vi "Main_v2.vi"() -> ()   [LabVIEW 2018, in "Application.lvlib"]
doc: "This VI is the main application VI in the Delacor QMH project template. This application VI is implemented as a simple state machine, which communicates with two different Delacor QMH modules.\n_____\nBased on DQMH Project Template 6.0.0.91."
uses:
  Application.lvlib
  type defs/HW config.ctl
  eMIC response.ctl
  Application Data--cluster.ctl
  DRV cluster.ctl
  App States.ctl
  eMICs Cluster.ctl
  Switches Module/MB switches Module.lvlib
  CE14 eMIC module/CE14 eMIC module.lvlib
  MB 01 switches Module/MB 01 switches Module.lvlib
  DMM Module/DMM Module.lvlib
  CE14  Module/CE14  Module.lvlib
panel:
  out "eMIC response":T1
  out "HV60D button":refnum<vi>[](array[refnum])
  out "HW config":T2={"DMM"="COM15", "mux"="COM11", "demux"="COM16", "eMIC1"="COM13", "eMIC2"="COM6", "eMIC3"="COM9", "eMIC4"="COM10", "eMIC5"="COM12", "eMIC6"="COM11"}
  out "CE14 Module Running?":bool
  in  "Read ACI, ACV  from  eMIC(x6)":bool
  out "DCI":dbl
  out "DCV":dbl
  in  "Sets to Display":u16(ring)=2 items=["1st Display", "2nd Display", "1st & 2nd Display"]
  in  "Read DCI, DCV  from DMM":bool
  in  "Detector Rate":u8(ring)=2 items=["SLOW", "MID", "FAST"]
  in  "DCI range":dbl=10.0
  in  "DCV range":dbl=1000.0
  in  "config DMM":bool
  in  "mux2-1(DMM I) encode":enum16{"DMM I (0.5)", "DMM I (12)"}(ring)
  in  "DMM input Selection":bool
  in  "mux6_1(3wires)_encode":T3(ring)
  in  "mux6-1(x1)":bool
  in  "Time duration(ms)":i32
  in  "mux10_1(x6)_encode":T4(ring)
  in  "mux10-1(x6)":bool
  in  "eMIC (x6)":bool[](array[boolean])=[FALSE, FALSE, FALSE, FALSE, FALSE, FALSE]
  in  "eMIC":bool
  in  "demux1_10(x6)":T5(ring)
  in  "demux1-10(x6)":bool
  in  "SC enable":bool=TRUE
  in  "SC Enable":bool
  in  "M054 Close":bool
  in  "Arduino Close":bool
  in  "DMM Close":bool
  in  "M054 name":refnum<visa-resource-name>="COM11"
  in  "Arduino name":refnum<visa-resource-name>="COM16"
  in  "DMM name":refnum<visa-resource-name>="COM15"
  in  "M054 connect":bool
  in  "Arduino connect":bool
  in  "DMM connect":bool
  in  "Test":bool caption="Again"
  out "DMM Module Running?":bool
  out "MB01 Module Running?":bool
  in  "Start DMM Module Module":bool
  in  "Start MB01 Module Module":bool
  out "DRV 61":u32(colorbox)
  in  "Exit":bool
  in  "Pause":bool
  in  "Again":bool
  out "DRV 60":u32(colorbox) caption="60"
  out "DRV 59":u32(colorbox) caption="59"
  out "DRV 58":u32(colorbox) caption="58"
  out "DRV 57":u32(colorbox) caption="57"
  out "DRV 56":u32(colorbox) caption="56"
  out "DRV 55":u32(colorbox) caption="55"
  out "DRV 54":u32(colorbox) caption="54"
  out "DRV 53":u32(colorbox) caption="53"
  out "DRV 52":u32(colorbox) caption="52"
  out "DRV 51":u32(colorbox) caption="51"
  out "DRV 50":u32(colorbox) caption="50"
  out "DRV 49":u32(colorbox) caption="49"
  out "DRV 48":u32(colorbox) caption="48"
  out "DRV 47":u32(colorbox) caption="47"
  out "DRV 46":u32(colorbox) caption="46"
  out "DRV 45":u32(colorbox) caption="45"
  out "DRV 44":u32(colorbox) caption="44"
  out "DRV 43":u32(colorbox) caption="43"
  out "DRV 42":u32(colorbox) caption="42"
  out "DRV 41":u32(colorbox) caption="41"
  out "DRV 40":u32(colorbox) caption="40"
  out "DRV 39":u32(colorbox) caption="39"
  out "DRV 38":u32(colorbox) caption="38"
  out "DRV 37":u32(colorbox) caption="37"
  out "DRV 36":u32(colorbox) caption="36"
  out "DRV 35":u32(colorbox) caption="35"
  out "DRV 34":u32(colorbox) caption="34"
  out "DRV 33":u32(colorbox) caption="33"
  out "DRV 32":u32(colorbox) caption="32"
  out "DRV 31":u32(colorbox) caption="31"
  out "DRV 30":u32(colorbox) caption="30"
  out "DRV 29":u32(colorbox) caption="29"
  out "DRV 28":u32(colorbox) caption="28"
  out "DRV 27":u32(colorbox) caption="27"
  out "DRV 26":u32(colorbox) caption="26"
  out "DRV 25":u32(colorbox) caption="25"
  out "DRV 24":u32(colorbox) caption="24"
  out "DRV 23":u32(colorbox) caption="23"
  out "DRV 22":u32(colorbox) caption="22"
  out "DRV 21":u32(colorbox) caption="21"
  out "DRV 20":u32(colorbox) caption="20"
  out "DRV 19":u32(colorbox)=4375612 caption="19"
  out "DRV 18":u32(colorbox) caption="18"
  out "DRV 17":u32(colorbox) caption="17"
  out "DRV 16":u32(colorbox) caption="16"
  out "DRV 15":u32(colorbox) caption="15"
  out "DRV 14":u32(colorbox) caption="14"
  out "DRV 13":u32(colorbox)=4375612 caption="13"
  out "DRV 12":u32(colorbox) caption="12"
  out "DRV 11":u32(colorbox) caption="11"
  out "DRV 10":u32(colorbox) caption="10"
  out "DRV 9":u32(colorbox) caption="9"
  out "DRV 8":u32(colorbox) caption="8"
  out "DRV 7":u32(colorbox)=4375612 caption="7"
  out "DRV 6":u32(colorbox) caption="6"
  out "DRV 5":u32(colorbox) caption="5"
  out "DRV 4":u32(colorbox) caption="4"
  out "DRV 3":u32(colorbox) caption="3"
  out "DRV 2":u32(colorbox) caption="2"
  out "DRV 1":u32(colorbox)=13224393 caption="1"
  out "version":string caption="Version"
  in  "Hide Switches Module Module":bool
  in  "Show Switches Module Module":bool
  in  "Hide CE14 eMIC module Module":bool
  in  "Show CE14 eMIC module Module":bool
  in  "Stop CE14 eMIC module Module":bool
  in  "Stop Switches Module Module":bool
  in  "Start Switches Module Module":bool
  out "Active CE14 eMIC module Modules":string[](array[string])
  in  "Start New Instance CE14 eMIC module Module":bool
  in  "Select CE14 eMIC module Module Instance":i32(ring)=-1 items=["All"=-1, "1"=1, "2"=2, "3"=3, "4"=4, "5"=5, "6"=6]
  in  "Switches Module Module: Do Something Else":dbl caption="Do Something Else"
  in  "Switches Module Module: Do Something":bool
  out "Switches Module Running?":bool
  out "Status":string
  # "HV-60D: LED POWER DRIVER ON-LINE TESTER"
  # "DCI range:  10mV; 100mV;  1A, 10A"
  # "DCV range: 100mV/1V; 10V, 1000V"
  # "This top-level application allows you to launch and control a singleton module, and multiple instances of a cloneable module."
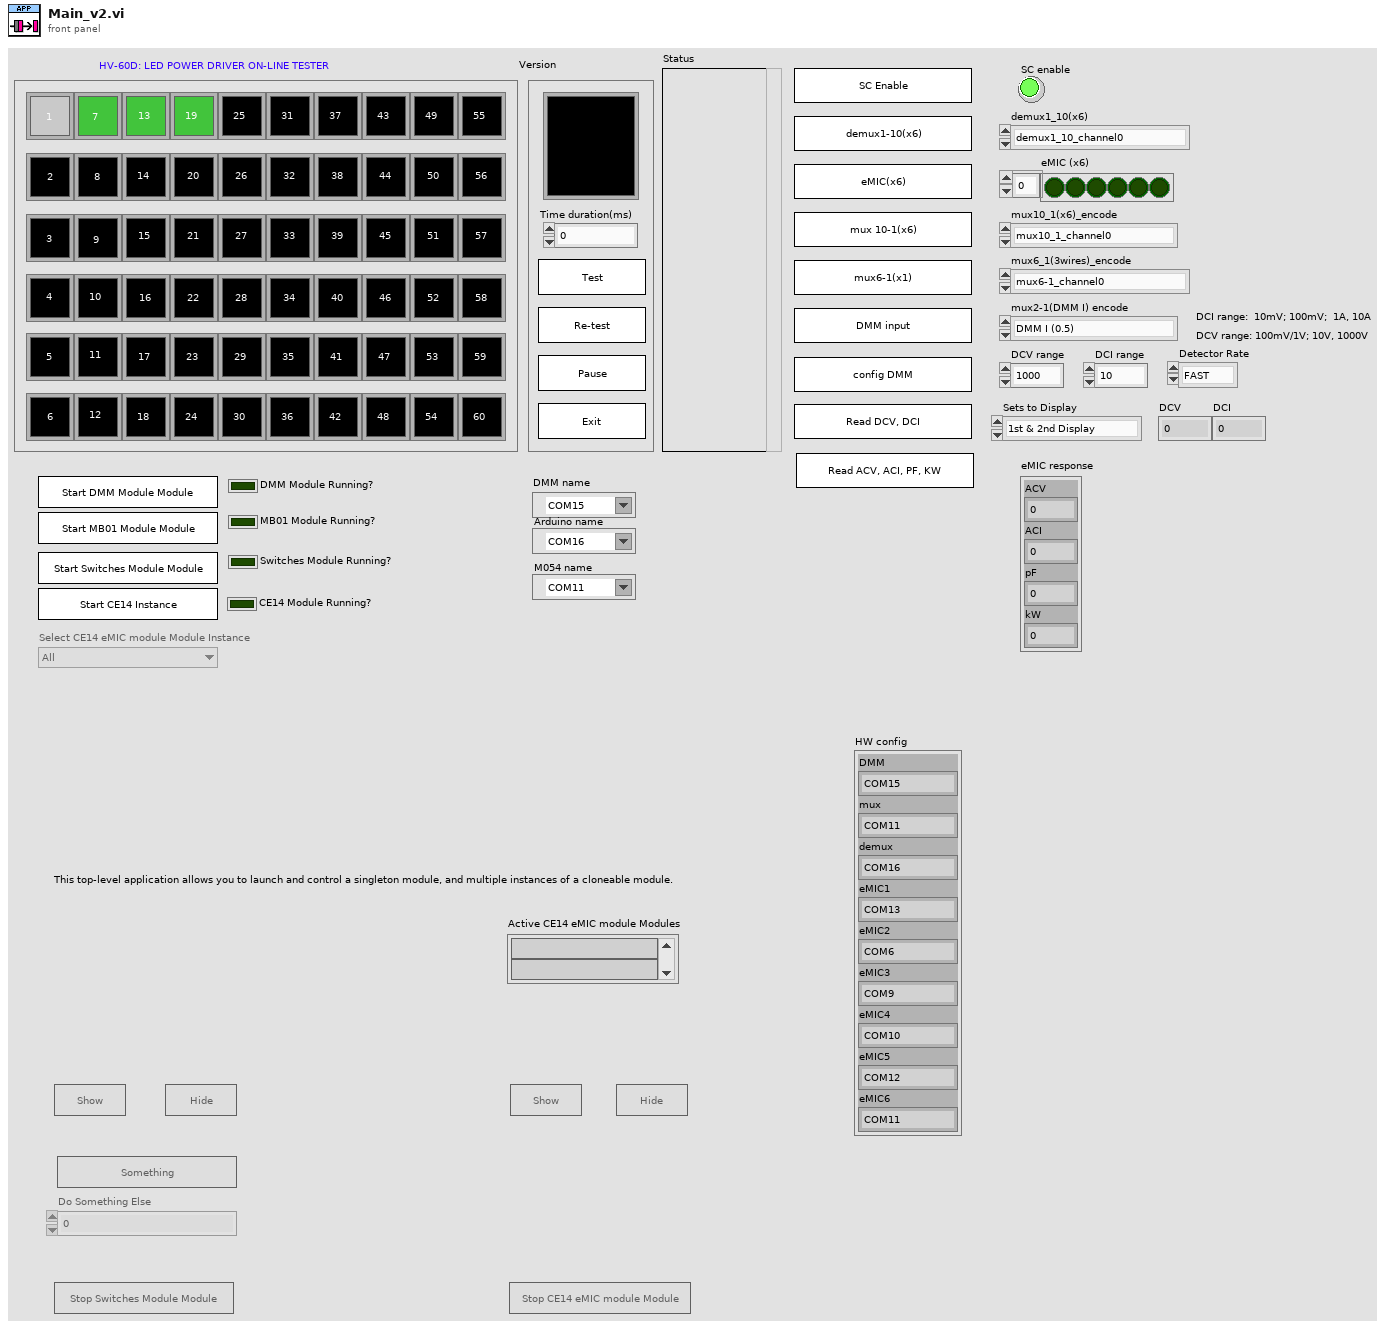
[diagram p1: front panel]
types:
  T1 = typedef "Application.lvlib/eMIC response.ctl" = cluster{"ACV":dbl, "ACI":dbl, "pF":dbl, "kW":dbl}
  T2 = typedef "Application.lvlib/HW config.ctl" = cluster{"DMM":string, "mux":string, "demux":string, "eMIC1":string, "eMIC2":string, "eMIC3":string, "eMIC4":string, "eMIC5":string, "eMIC6":string}
  T3 = enum16{"mux6-1_channel0", "mux6_1_channel1_0", "mux6_1_channel1_1", "mux6-1_channel1_2", "mux6_1_channel1_3", "mux6_1_channel2_0", "mux6_1_channel2_1", "mux6_1_channel2_2", "mux6_1_channel2_3", "mux6_1_channel3_0", "mux6_1_channel3_1", "mux6_1_channel3_2", "mux6_1_channel3_3", "mux6_1_channel4_0", "mux6_1_channel4_1", "mux6_1_channel4_2", "mux6_1_channel4_3", "mux6_1_channel5_0", "mux6_1_channel5_1", "mux6_1_channel5_2", "mux6_1_channel5_3", "mux6_1_channel6_0", "mux6_1_channel6_1", "mux6_1_channel6_2", "mux6_1_channel6_3"}
  T4 = enum16{"mux10_1_channel0", "mux10_1_channel1", "mux10_1_channel2", "mux10_1_channel3", "mux10_1_channel4", "mux10_1_channel5", "mux10_1_channel6", "mux10_1_channel7", "mux10_1_channel8", "mux10_1_channel9", "mux10_1_channel10"}
  T5 = enum16{"demux1_10_channel0", "demux1_10_channel1", "demux1_10_channel2", "demux1_10_channel3", "demux1_10_channel4", "demux1_10_channel5", "demux1_10_channel6", "demux1_10_channel7", "demux1_10_channel8", "demux1_10_channel9", "demux1_10_channel10"}
  T6 = typedef "Application.lvlib/App States.ctl" = enum16{"Apps.Initialize0", "Apps.Initialize1", "Apps.Initialize2", "Apps.Initialize3", "Apps.Initialize4", "Apps.Initialize Panel", "Apps.UI Interlocks", "Apps.UI.Reinitiatize", "Apps.Update Status", "Apps.Wait for Event", "Apps.Exit"}
  T7 = typedef "Application.lvlib/Application Data--cluster.ctl" = cluster{"Status":string, "Singleton Controls":refnum<vi>[], "Cloneable Controls":refnum<vi>[], "Module Ring Value":i32, "HW config":T2, "DUT values":T8[]}
  T8 = typedef "Application.lvlib/DRV cluster.ctl" = cluster{"Pass/Fail?":bool, "AC Characteristic":cluster{"Pass/Fail?":bool, "Voltage":cluster{"pass/fail?":bool, "Measured Value":dbl, "Upper Level":dbl, "Lower Level":dbl}, "Current":cluster{"pass/fail?":bool, "Measured Value":dbl, "Upper Level":dbl, "Lower Level":dbl}, "Power factor":cluster{"pass/fail?":bool, "Measured Value":dbl, "Upper Level":dbl, "Lower Level":dbl}, "Shorted Circuit":cluster{"Pass/Fail?":bool}}, "DC Characteristic":cluster{"Pass/Fail?":bool, "Voltage":cluster{"pass/fail?":bool, "Measured Value":dbl, "Upper Level":dbl, "Lower Level":dbl}, "Current":cluster{"pass/fail?":bool, "Measured Value":dbl, "Upper Level":dbl, "Lower Level":dbl}}}
  T9 = typedef "CE14  Module.lvlib/Broadcast Events--cluster.ctl" = cluster{"Module Did Init":refnum<user-event>, "Status Updated":refnum<user-event>, "Error Reported":refnum<user-event>, "Module Did Stop":refnum<user-event>, "Update Module Execution Status":refnum<user-event>, "eMICs response":refnum<user-event>}
  T10 = typedef "MB switches Module.lvlib/Broadcast Events--cluster.ctl" = cluster{"Module Did Init":refnum<user-event>, "Status Updated":refnum<user-event>, "Error Reported":refnum<user-event>, "Module Did Stop":refnum<user-event>, "Update Module Execution Status":refnum<user-event>}
  T11 = typedef "MB 01 switches Module.lvlib/Broadcast Events--cluster.ctl" = cluster{"Module Did Init":refnum<user-event>, "Status Updated":refnum<user-event>, "Error Reported":refnum<user-event>, "Module Did Stop":refnum<user-event>, "Update Module Execution Status":refnum<user-event>}
  T12 = typedef "DMM Module.lvlib/Broadcast Events--cluster.ctl" = cluster{"Module Did Init":refnum<user-event>, "Status Updated":refnum<user-event>, "Error Reported":refnum<user-event>, "Module Did Stop":refnum<user-event>, "Update Module Execution Status":refnum<user-event>}
  T13 = enum8{"Enabled", "Disabled", "Disabled and Grayed Out"}
  T14 = typedef "Application.lvlib/eMICs Cluster.ctl" = cluster{"eMIC 1":T1, "eMIC 2":T1, "eMIC 3":T1, "eMIC 4":T1, "eMIC 5":T1, "eMIC 6":T1}
  T15 = typedef "CE14_eMIC.lvlib/CE14.data.ctl" = cluster{"strings":string, "float":dbl, "Name":string}
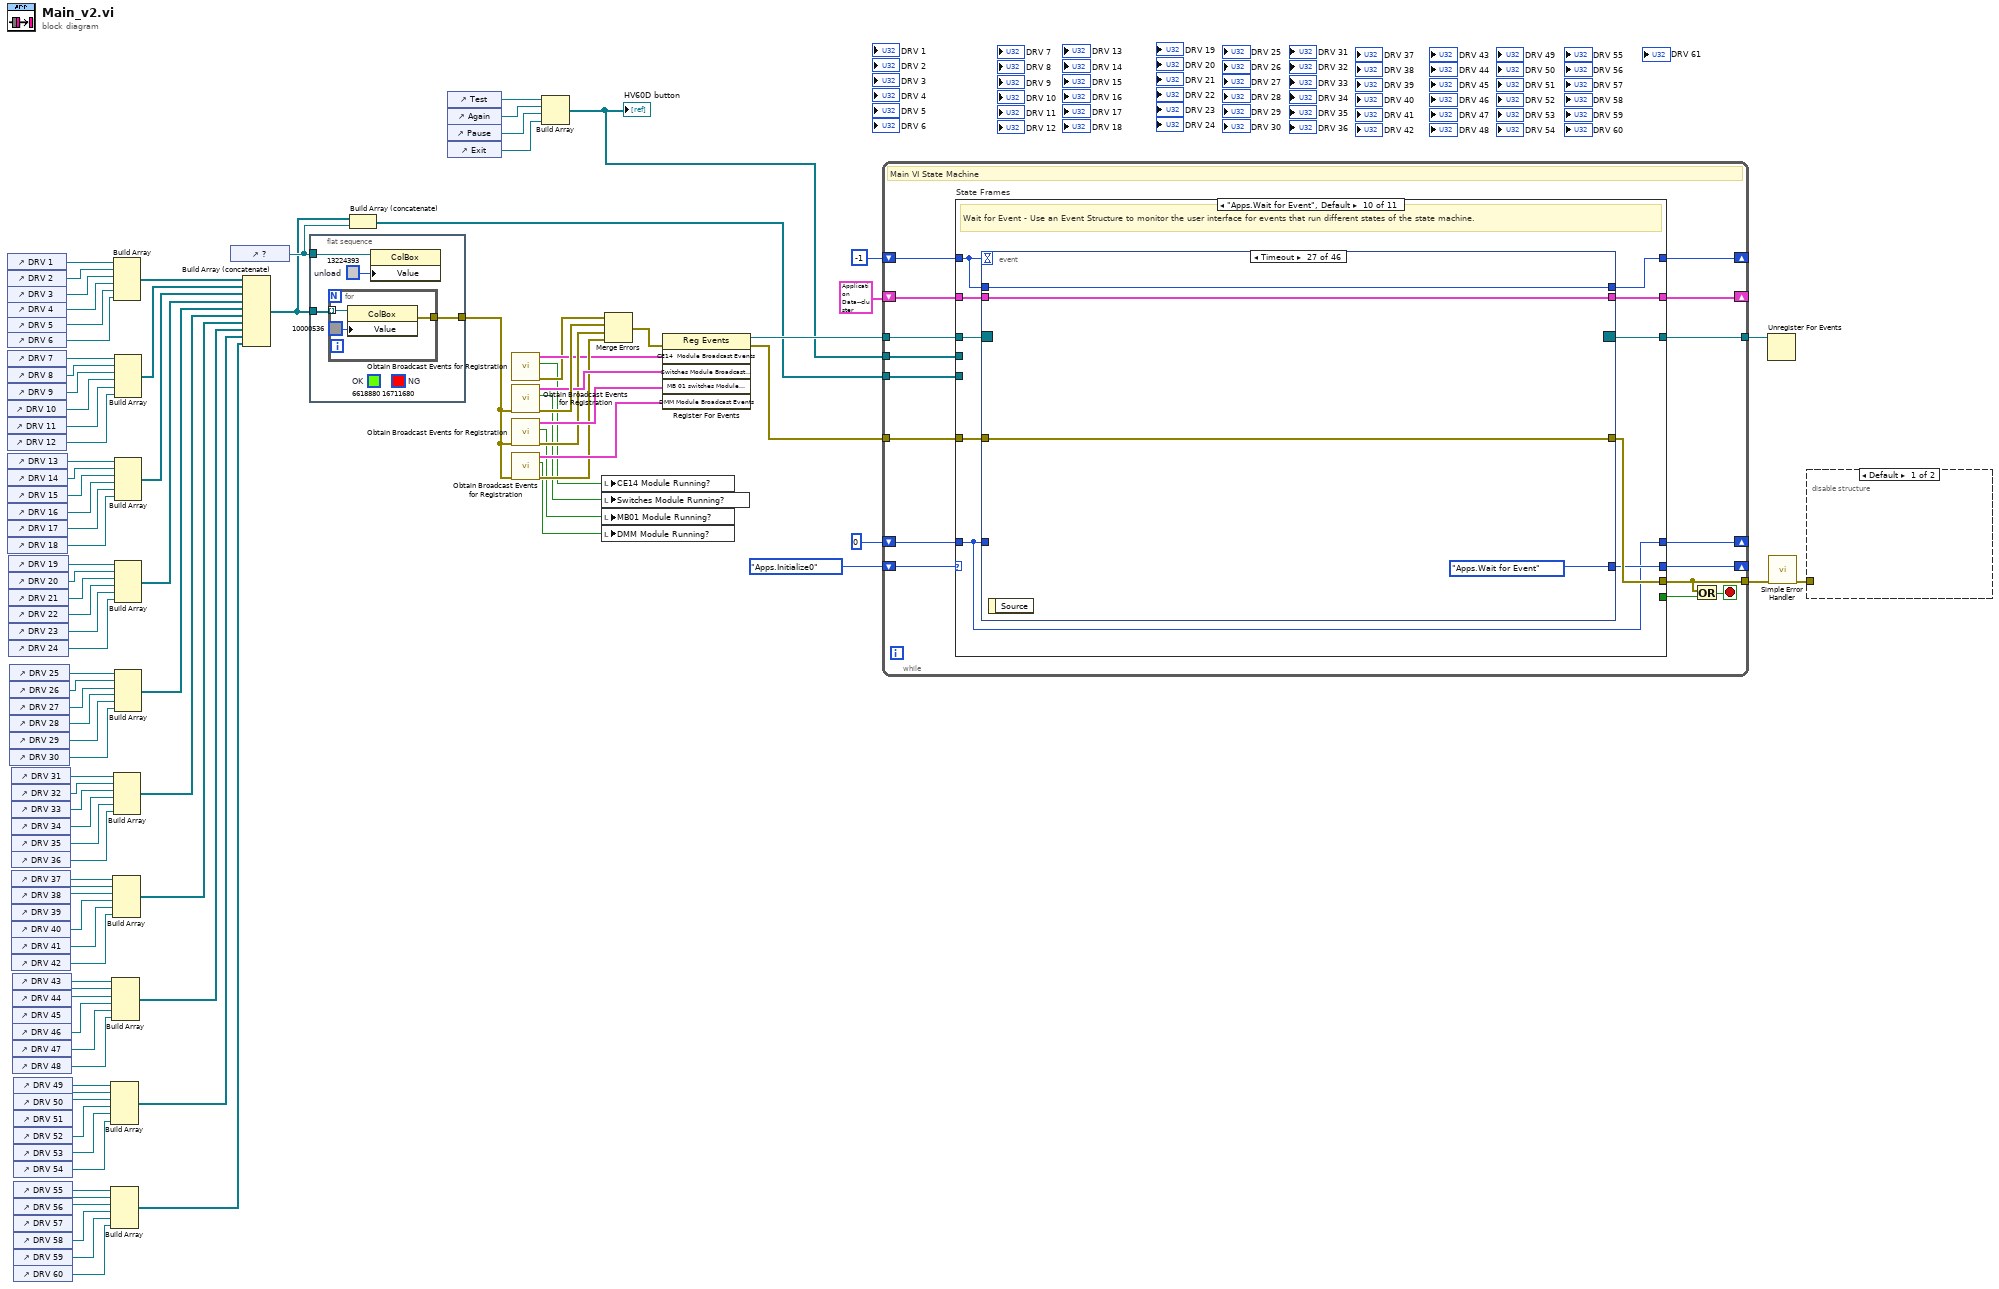
[diagram p0: block diagram]
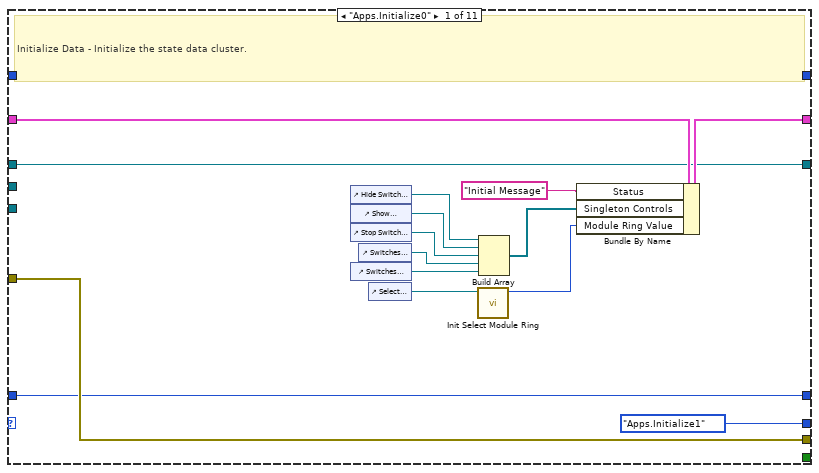
[diagram p2: hidden frame]
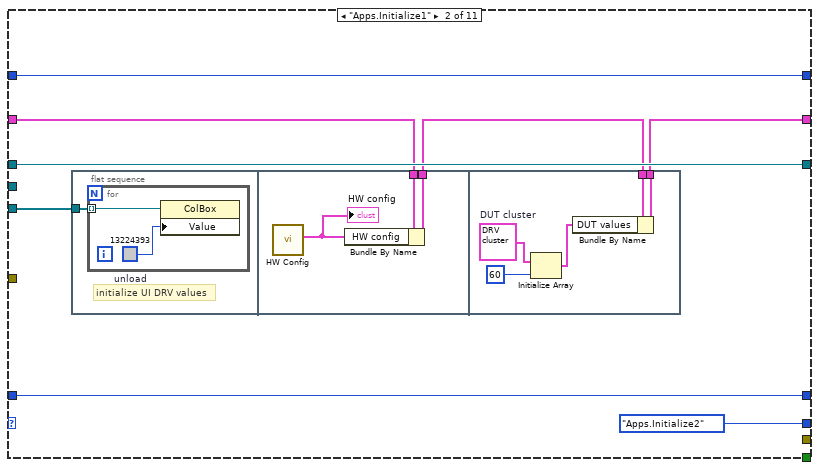
[diagram p3: hidden frame]
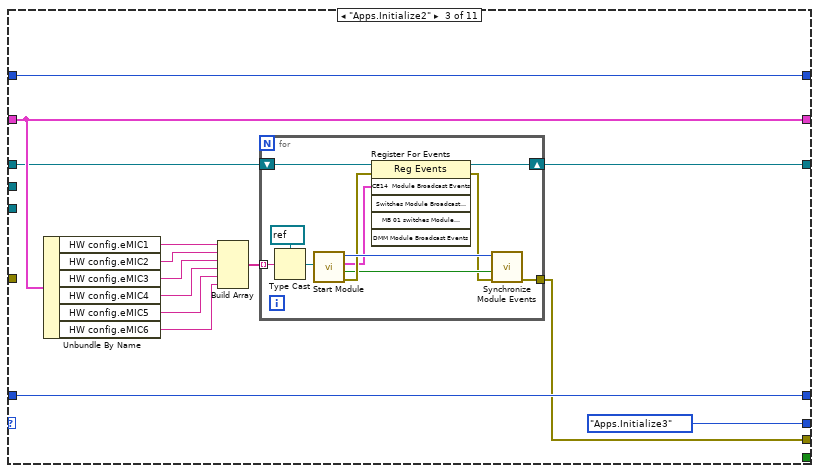
[diagram p4: hidden frame]
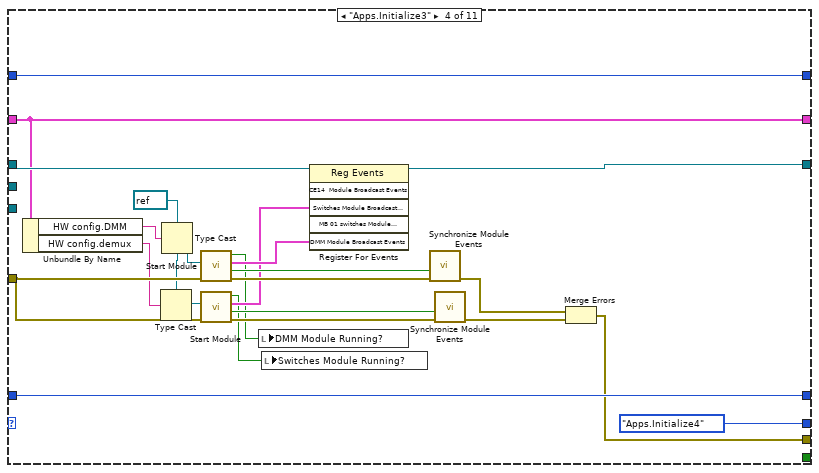
[diagram p5: hidden frame]
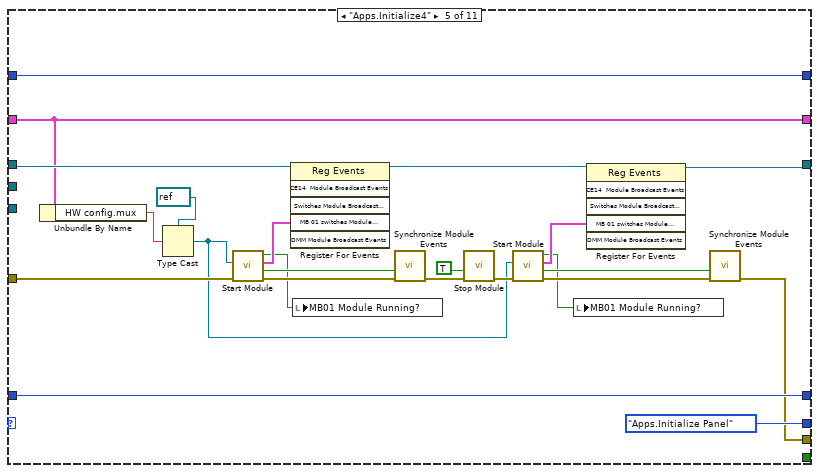
[diagram p6: hidden frame]
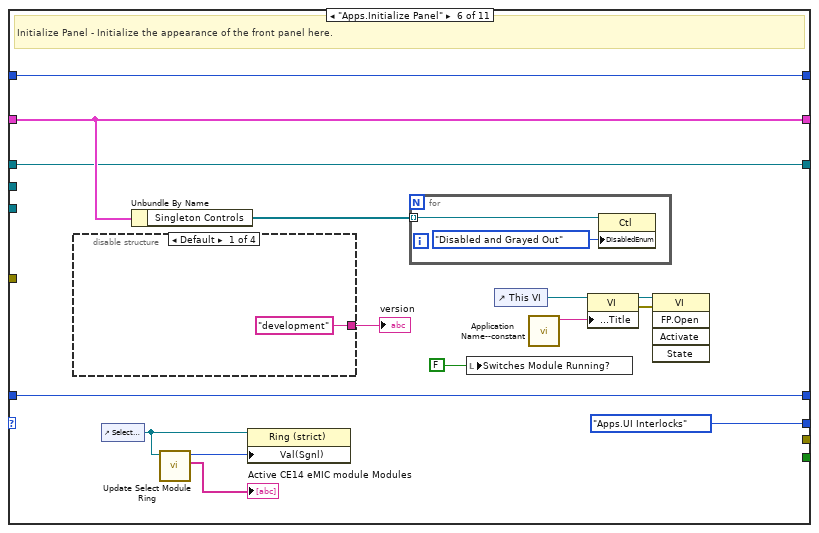
[diagram p7: hidden frame]
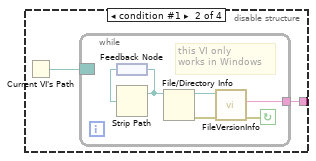
[diagram p8: hidden frame]
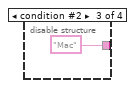
[diagram p9: hidden frame]
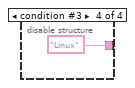
[diagram p10: hidden frame]
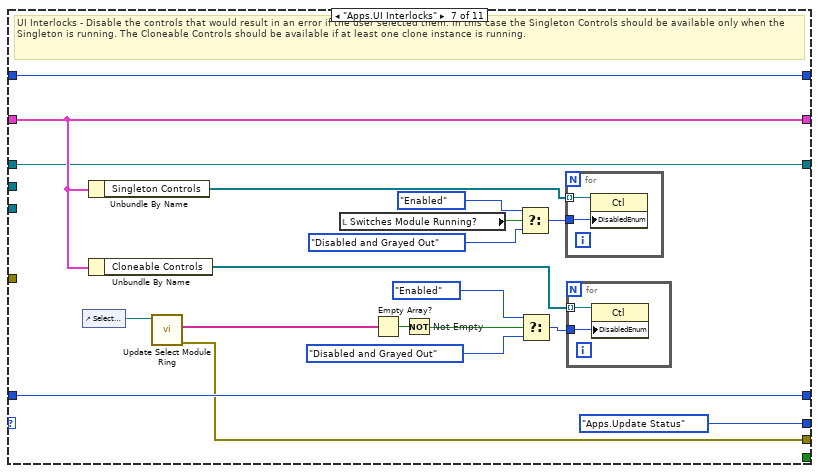
[diagram p11: hidden frame]
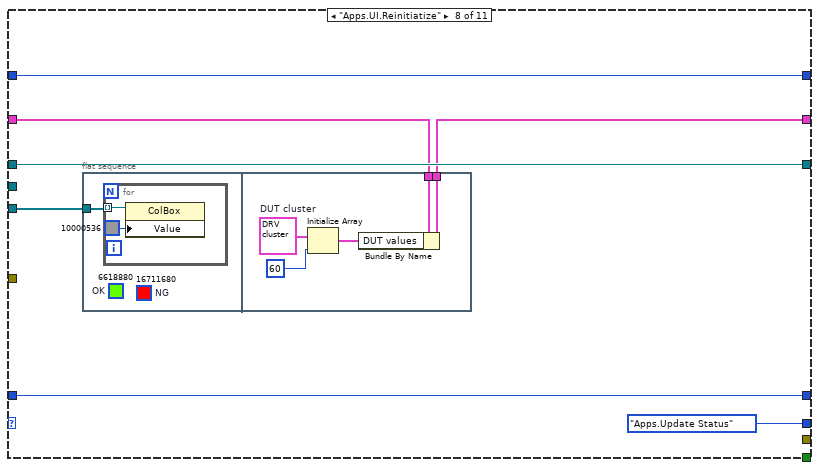
[diagram p12: hidden frame]
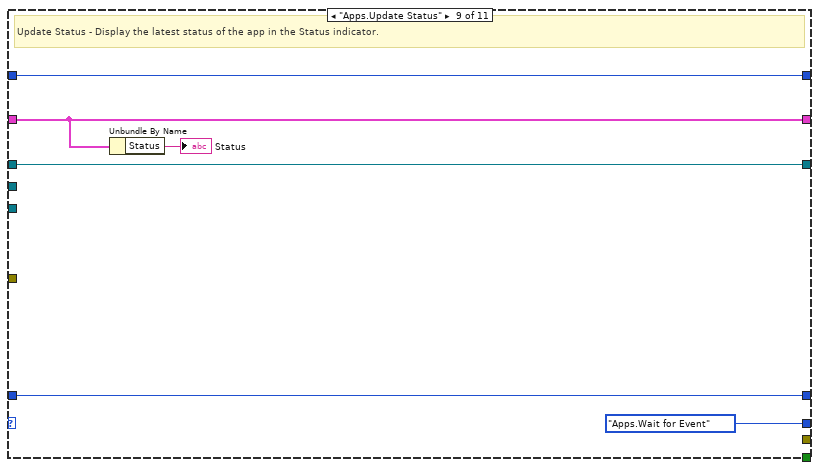
[diagram p13: hidden frame]
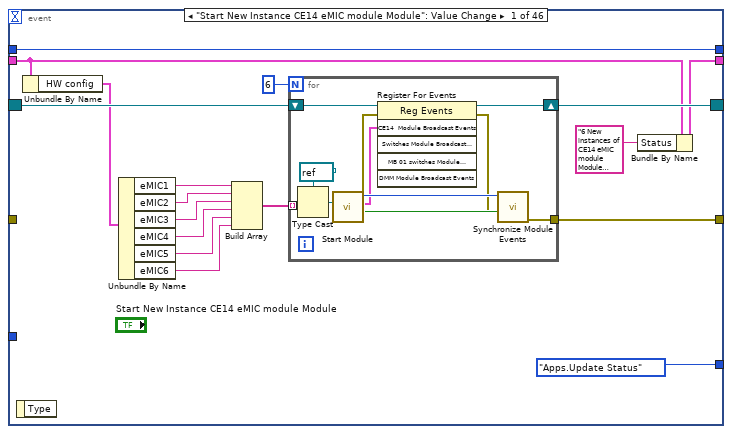
[diagram p14: hidden frame]
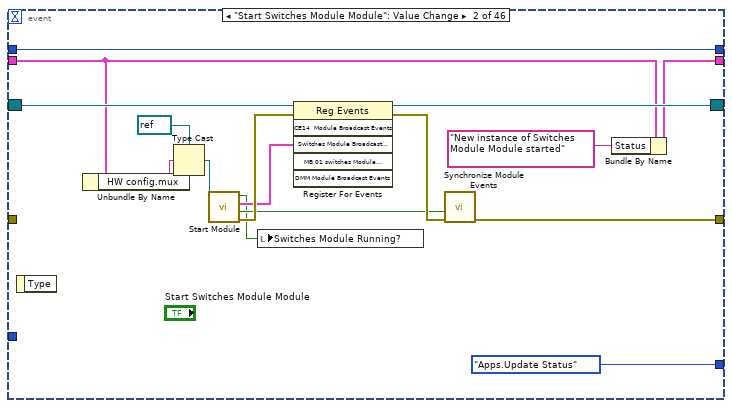
[diagram p15: hidden frame]
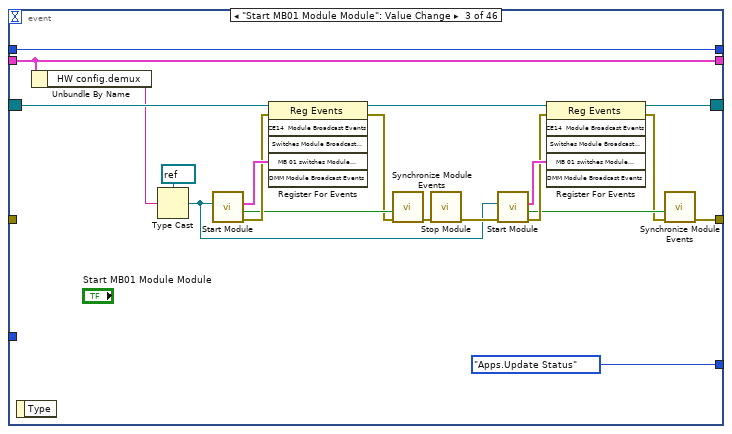
[diagram p16: hidden frame]
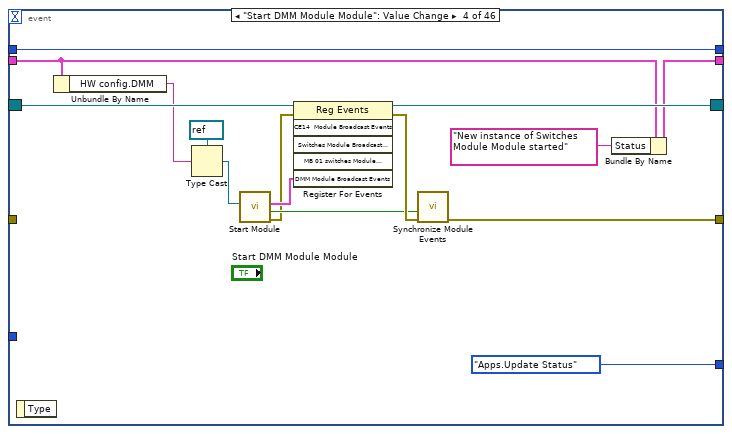
[diagram p17: hidden frame]
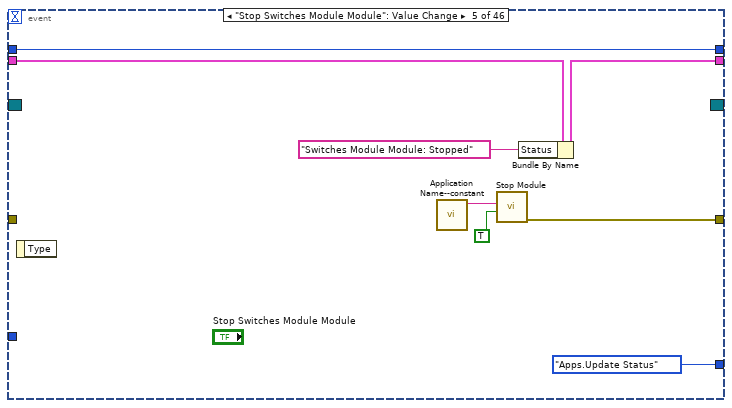
[diagram p18: hidden frame]
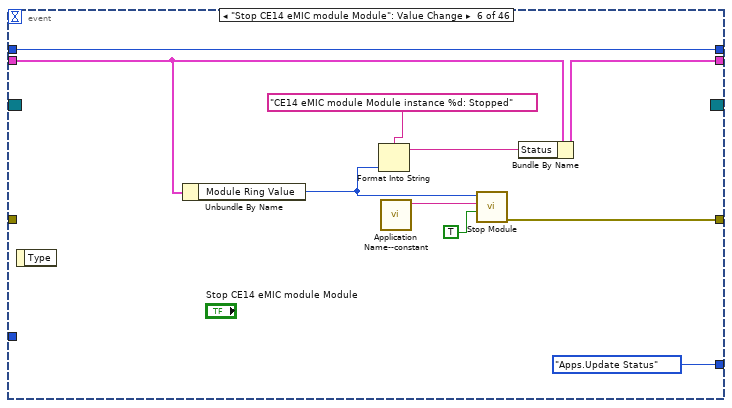
[diagram p19: hidden frame]
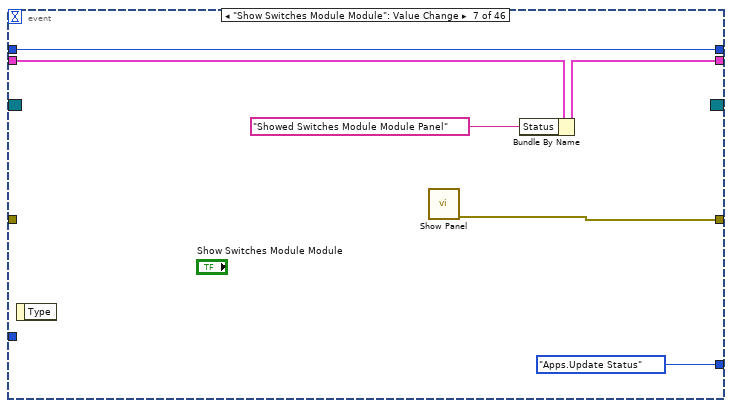
[diagram p20: hidden frame]
diagram:
  n1 = control-ref of="DRV 1"() -> (w92:refnum<vi>)
  n2 = control-ref of="DRV 2"() -> (w91:refnum<vi>)
  n3 = control-ref of="DRV 3"() -> (w90:refnum<vi>)
  n4 = control-ref of="DRV 4"() -> (w89:refnum<vi>)
  n5 = control-ref of="DRV 5"() -> (w88:refnum<vi>)
  n6 = control-ref of="DRV 6"() -> (w87:refnum<vi>)
  n7 = control-ref of="DRV 7"() -> (w81:refnum<vi>)
  n8 = control-ref of="DRV 8"() -> (w80:refnum<vi>)
  n9 = control-ref of="DRV 9"() -> (w79:refnum<vi>)
  n10 = control-ref of="DRV 10"() -> (w78:refnum<vi>)
  n11 = control-ref of="DRV 11"() -> (w77:refnum<vi>)
  n12 = control-ref of="DRV 12"() -> (w76:refnum<vi>)
  n13 = control-ref of="DRV 13"() -> (w70:refnum<vi>)
  n14 = control-ref of="DRV 14"() -> (w71:refnum<vi>)
  n15 = control-ref of="DRV 15"() -> (w72:refnum<vi>)
  n16 = control-ref of="DRV 16"() -> (w73:refnum<vi>)
  n17 = control-ref of="DRV 17"() -> (w74:refnum<vi>)
  n18 = control-ref of="DRV 18"() -> (w75:refnum<vi>)
  n19 = control-ref of="DRV 19"() -> (w69:refnum<vi>)
  n20 = control-ref of="DRV 20"() -> (w68:refnum<vi>)
  n21 = control-ref of="DRV 21"() -> (w67:refnum<vi>)
  n22 = control-ref of="DRV 22"() -> (w66:refnum<vi>)
  n23 = control-ref of="DRV 23"() -> (w65:refnum<vi>)
  n24 = control-ref of="DRV 24"() -> (w64:refnum<vi>)
  n25 = control-ref of="DRV 25"() -> (w58:refnum<vi>)
  n26 = control-ref of="DRV 26"() -> (w59:refnum<vi>)
  n27 = control-ref of="DRV 27"() -> (w60:refnum<vi>)
  n28 = control-ref of="DRV 28"() -> (w61:refnum<vi>)
  n29 = control-ref of="DRV 29"() -> (w62:refnum<vi>)
  n30 = control-ref of="DRV 30"() -> (w63:refnum<vi>)
  n31 = control-ref of="DRV 31"() -> (w57:refnum<vi>)
  n32 = control-ref of="DRV 32"() -> (w56:refnum<vi>)
  n33 = control-ref of="DRV 33"() -> (w55:refnum<vi>)
  n34 = control-ref of="DRV 34"() -> (w54:refnum<vi>)
  n35 = control-ref of="DRV 35"() -> (w53:refnum<vi>)
  n36 = control-ref of="DRV 36"() -> (w52:refnum<vi>)
  n37 = control-ref of="DRV 37"() -> (w46:refnum<vi>)
  n38 = control-ref of="DRV 38"() -> (w47:refnum<vi>)
  n39 = control-ref of="DRV 39"() -> (w48:refnum<vi>)
  n40 = control-ref of="DRV 40"() -> (w49:refnum<vi>)
  n41 = control-ref of="DRV 41"() -> (w50:refnum<vi>)
  n42 = control-ref of="DRV 42"() -> (w51:refnum<vi>)
  n43 = control-ref of="DRV 43"() -> (w45:refnum<vi>)
  n44 = control-ref of="DRV 44"() -> (w44:refnum<vi>)
  n45 = control-ref of="DRV 45"() -> (w43:refnum<vi>)
  n46 = control-ref of="DRV 46"() -> (w42:refnum<vi>)
  n47 = control-ref of="DRV 47"() -> (w41:refnum<vi>)
  n48 = control-ref of="DRV 48"() -> (w40:refnum<vi>)
  n49 = control-ref of="DRV 49"() -> (w34:refnum<vi>)
  n50 = control-ref of="DRV 50"() -> (w35:refnum<vi>)
  n51 = control-ref of="DRV 51"() -> (w36:refnum<vi>)
  n52 = control-ref of="DRV 52"() -> (w37:refnum<vi>)
  n53 = control-ref of="DRV 53"() -> (w38:refnum<vi>)
  n54 = control-ref of="DRV 54"() -> (w39:refnum<vi>)
  n55 = control-ref of="DRV 55"() -> (w33:refnum<vi>)
  n56 = control-ref of="DRV 56"() -> (w32:refnum<vi>)
  n57 = control-ref of="DRV 57"() -> (w31:refnum<vi>)
  n58 = control-ref of="DRV 58"() -> (w30:refnum<vi>)
  n59 = control-ref of="DRV 59"() -> (w29:refnum<vi>)
  n60 = control-ref of="DRV 60"() -> (w28:refnum<vi>)
  n61 = Build Array(w34, w35, w36, w37, w38, w39) -> (w19:refnum<vi>[])
  n62 = Build Array(w33, w32, w31, w30, w29, w28) -> (w18:refnum<vi>[])
  n63 = Build Array(w45, w44, w43, w42, w41, w40) -> (w20:refnum<vi>[])
  n64 = Build Array(w46, w47, w48, w49, w50, w51) -> (w21:refnum<vi>[])
  n65 = Build Array(w92, w91, w90, w89, w88, w87) -> (w27:refnum<vi>[])
  n66 = Build Array(w57, w56, w55, w54, w53, w52) -> (w22:refnum<vi>[])
  n67 = Build Array(w81, w80, w79, w78, w77, w76) -> (w26:refnum<vi>[])
  n68 = Build Array(w70, w71, w72, w73, w74, w75) -> (w25:refnum<vi>[])
  n69 = Build Array(w69, w68, w67, w66, w65, w64) -> (w24:refnum<vi>[])
  n70 = Build Array(w58, w59, w60, w61, w62, w63) -> (w23:refnum<vi>[])
  n71 = control-ref of="?"() -> (w8:refnum<vi>)
  n72 = Build Array (concatenate)(w27, w26, w25, w24, w23, w22, w21, w20, w19, w18) -> (w7:refnum<vi>[])
  n73 = flat-sequence {
    tunnel: w7 -> [w105]
    tunnel: [w104] -> w17
    tunnel: w8 -> [w102]
    frame #0 {
      (unwired) u32 16711680  # NG
      (unwired) u32 6618880  # OK
      w103 = u32 13224393  # unload
      n74 = for {
        tunnel: w105 -> [w107] mode=indexing
        tunnel: [w106] -> w104
        n75 = property class="ColBox"(reference=w107, "Value"=u32 10000536 ("DRV 1")) -> (error out=w106:errorcluster)  [unwired: 1 in, 1 out]
      }
      n76 = property class="ColBox"(reference=w102, "Value"=w103) -> ()  [unwired: 1 in, 2 out]
    }
  }
  n77 = Build Array (concatenate)(w7, w8) -> (w6:refnum<vi>[])
  n78 = control-ref of="Test"() -> (w5:refnum<vi>)
  n79 = control-ref of="Again"() -> (w4:refnum<vi>)
  n80 = control-ref of="Pause"() -> (w3:refnum<vi>)
  n81 = control-ref of="Exit"() -> (w2:refnum<vi>)
  n82 = call "Obtain Broadcast Events for Registration.vi"() -> ("error out"=w14:errorcluster, "Already running?"=w12:bool, "CE14  Module Broadcast Events"=w15:T9)  [unwired: 9 in]
  n83 = call "Obtain Broadcast Events for Registration.vi"("error in (no error)"=w17) -> ("error out"=w98:errorcluster, "Already running?"=w13:bool, "Switches Module Broadcast Events"=w96:T10)  [unwired: 8 in]
  n84 = call "Obtain Broadcast Events for Registration.vi"("error in (no error)"=w17) -> ("error out"=w85:errorcluster, "Already running?"=w10:bool, "MB 01 switches Module Broadcast Events"=w86:T11)  [unwired: 8 in]
  n85 = call "Obtain Broadcast Events for Registration.vi"("error in (no error)"=w17) -> ("error out"=w83:errorcluster, "Already running?"=w11:bool, "DMM Module Broadcast Events"=w84:T12)  [unwired: 8 in]
  n86 = Build Array(w5, w4, w3, w2) -> (w1:refnum<vi>[])
  "HV60D button" <- w1
  n87 = local write "CE14 Module Running?"(w12) -> ()
  n88 = local write "Switches Module Running?"(w13) -> ()
  n89 = local write "MB01 Module Running?"(w10) -> ()
  n90 = local write "DMM Module Running?"(w11) -> ()
  n91 = Merge Errors(w14, w98, w85, w83) -> (w99:errorcluster)
  n92 = register-events(error in=w99, w15, w96, w86, w84) -> (reference out=w93:refnum<event-registration>, error out=w9:errorcluster)  [unwired: 1 in]
  n93 = while {
    shift-right: [w121] -> _
    shift-left: T7 {"Status"="", "Singleton Controls"=[], "Cloneable Controls"=[], "Module Ring Value"=0, "HW config"={"DMM"="COM15", "mux"="COM11", "demux"="COM16", "eMIC1"="COM13", "eMIC2"="COM6", "eMIC3"="COM9", "eMIC4"="COM10", "eMIC5"="COM12", "eMIC6"="COM11"}, "DUT values"=[]} ("Data Cluster") -> [w122]
    tunnel: [w124] -> w101
    shift-right: [w117] -> _
    shift-left: App_States."Apps.Initialize0" ("Initial State") -> [w119]
    tunnel: w9 -> [w123]
    tunnel: w93 -> [w116]
    tunnel: [w115] -> w94
    shift-right: [w113] -> _
    shift-left: 0 -> [w114]
    shift-right: [w111] -> _
    shift-left: -1 -> [w112]
    tunnel: w6 -> [w110]
    tunnel: w1 -> [w109]
    stop <- w118 stop-if-true
    # "Main VI State Machine"
    n94 = case "State Frames" shown="\"Apps.Wait for Event\", Default" w119 {
      tunnel: [w140 _ w160 w193 w214 _ w259 _ _ w312 w714] -> w124
      tunnel: w122 -> [w139 w143 w170 w190 w211 w243 w268 w282 w302 w309 w712]
      tunnel: [w138 w142 w170 w190 w211 w243 w268 w283 w302 w308 w712] -> w121
      tunnel: [_ _ _ _ _ _ _ _ _ _ w711] -> w120
      tunnel: [App_States."Apps.Initialize1" ("State") App_States."Apps.Initialize2" ("State") App_States."Apps.Initialize3" ("State") App_States."Apps.Initialize4" ("State") App_States."Apps.Initialize Panel" ("State") App_States."Apps.UI Interlocks" ("State") App_States."Apps.Update Status" ("State") App_States."Apps.Update Status" ("State") App_States."Apps.Wait for Event" ("State") w307 App_States."Apps.Exit" ("State")] -> w117
      tunnel: w116 -> [w129 w148 w162 w203 w226 w240 w264 w288 w299 w311 w709]
      tunnel: [w129 w148 w161 w204 w218 w240 w264 w288 w299 w310 w709] -> w115
      tunnel: w123 -> [w140 _ _ w196 w227 _ _ _ _ w306 _]
      tunnel: w114 -> [w128 w147 w173 w207 w230 w236 w263 w287 w298 w305 w706]
      tunnel: [w128 w147 w173 w207 w230 w236 w263 w287 w298 w305 w706] -> w113
      tunnel: w112 -> [w127 w146 w172 w206 w229 w234 w262 w286 w297 w304 w705]
      tunnel: [w127 w146 w172 w206 w229 w234 w262 w286 w297 w303 w705] -> w111
      tunnel: w110 -> [_ w144 _ _ _ _ _ w285 _ _ _]
      tunnel: w109 -> [_ _ _ _ _ _ _ _ _ _ _]
      frame "Apps.Initialize0" {
        # "Initialize Data - Initialize the state data cluster."
        n95 = control-ref of="Hide Switches Module Module"() -> (w136:refnum<vi>)
        n96 = control-ref of="Show Switches Module Module"() -> (w135:refnum<vi>)
        n97 = control-ref of="Stop Switches Module Module"() -> (w134:refnum<vi>)
        n98 = control-ref of="Switches Module Module: Do Something"() -> (w132:refnum<vi>)
        n99 = control-ref of="Switches Module Module: Do Something Else"() -> (w133:refnum<vi>)
        n100 = control-ref of="Select CE14 eMIC module Module Instance"() -> (w126:refnum<vi>)
        n101 = call "Init Select Module Ring.vi"("Select Module Ring Ref"=w126) -> ("Value for All Modules"=w125:i32)  [unwired: 8 in, 2 out]
        n102 = Build Array(w136, w135, w134, w133, w132) -> (w131:refnum<vi>[])
        n103 = Bundle By Name(cluster=w139, "Status"="Initial Message" ("Initial Message"), "Singleton Controls"=w131, "Module Ring Value"=w125) -> (w138:T7)
      }
      frame "Apps.Initialize1" {
        n104 = flat-sequence {
          tunnel: w144 -> [w149]
          tunnel: w143 -> [w153]
          tunnel: [w152] -> w141
          tunnel: [w156] -> w142
          tunnel: w141 -> [w155]
          frame #0 {
            # "initialize UI DRV values"
            n105 = for {
              tunnel: w149 -> [w151] mode=indexing
              w150 = u32 13224393  # unload
              n106 = property class="ColBox"(reference=w151, "Value"=w150) -> ()  [unwired: 1 in, 2 out]
            }
          }
          frame #1 {
            n107 = call "HW Config.vi"() -> ("HW config 2"=w154:T2)  [unwired: 10 in, 1 out]
            "HW config" <- w154
            n108 = Bundle By Name(cluster=w153, "HW config"=w154) -> (w152:T7)
          }
          frame #2 {
            w159 = T8 {"Pass/Fail?"=FALSE, "AC Characteristic"={"Pass/Fail?"=FALSE, "Voltage"={"pass/fail?"=FALSE, "Measured Value"=0.0, "Upper Level"=0.0, "Lower Level"=0.0}, "Current"={"pass/fail?"=FALSE, "Measured Value"=0.0, "Upper Level"=0.0, "Lower Level"=0.0}, "Power factor"={"pass/fail?"=FALSE, "Measured Value"=0.0, "Upper Level"=0.0, "Lower Level"=0.0}, "Shorted Circuit"={"Pass/Fail?"=FALSE}}, "DC Characteristic"={"Pass/Fail?"=FALSE, "Voltage"={"pass/fail?"=FALSE, "Measured Value"=0.0, "Upper Level"=0.0, "Lower Level"=0.0}, "Current"={"pass/fail?"=FALSE, "Measured Value"=0.0, "Upper Level"=0.0, "Lower Level"=0.0}}}  # DUT cluster
            n109 = Initialize Array(w159, 60 ("dimension size")) -> (w157:T8[])
            n110 = Bundle By Name(cluster=w155, "DUT values"=w157) -> (w156:T7)
          }
        }
      }
      frame "Apps.Initialize2" {
        n111 = Unbundle By Name(w170) -> ("HW config.eMIC1"=w169:string, "HW config.eMIC2"=w168:string, "HW config.eMIC3"=w167:string, "HW config.eMIC4"=w166:string, "HW config.eMIC5"=w165:string, "HW config.eMIC6"=w164:string)
        n112 = Build Array(w169, w168, w167, w166, w165, w164) -> (w163:string[])
        n113 = for {
          tunnel: [w177] -> w160
          shift-right: [w183] -> w161
          shift-left: w162 -> [w184]
          tunnel: w163 -> [w175] mode=indexing
          n114 = Type Cast(type=refnum<visa-resource-name> refnum ("VISA resource name"), x=w175) -> (*(type *) &x=w174:refnum<visa-resource-name>)
          n115 = call "Start Module.vi"("VISA resource name"=w174) -> ("error out"=w181:errorcluster, "Wait for Event Sync?"=w179:bool, "CE14  Module Broadcast Events"=w180:T9, "Module ID"=w182:i32)  [unwired: 7 in]
          n116 = register-events(reference=w184, error in=w181, w180) -> (reference out=w183:refnum<event-registration>, error out=w178:errorcluster)  [unwired: 3 in]
          n117 = call "Synchronize Module Events.vi"("error in"=w178, "Wait for Event Sync?"=w179, "Module ID in"=w182) -> ("error out"=w177:errorcluster)  [unwired: 7 in, 1 out]
        }
      }
      frame "Apps.Initialize3" {
        w186 = refnum<visa-resource-name> refnum ("VISA resource name 2")
        n118 = Unbundle By Name(w190) -> ("HW config.DMM"=w189:string, "HW config.demux"=w187:string)
        n119 = Type Cast(type=w186, x=w187) -> (*(type *) &x=w185:refnum<visa-resource-name>)
        n120 = Type Cast(type=w186, x=w189) -> (*(type *) &x=w188:refnum<visa-resource-name>)
        n121 = call "Start Module.vi"("error in (no error)"=w196, "VISA resource name 2"=w188) -> ("error out"=w200:errorcluster, "Wait for Event Sync?"=w202:bool, "DMM Module Broadcast Events"=w201:T12, "Module Was Already Running?"=w192:bool)  [unwired: 6 in]
        n122 = call "Start Module.vi"("error in (no error)"=w196, "VISA resource name"=w185) -> ("error out"=w197:errorcluster, "Wait for Event Sync?"=w198:bool, "Switches Module Broadcast Events"=w199:T10, "Module Was Already Running?"=w191:bool)  [unwired: 6 in]
        n123 = local write "DMM Module Running?"(w192) -> ()
        n124 = local write "Switches Module Running?"(w191) -> ()
        n125 = register-events(reference=w203, w199, w201) -> (reference out=w204:refnum<event-registration>)  [unwired: 3 in, 1 out]
        n126 = call "Synchronize Module Events.vi"("error in"=w200, "Wait for Event Sync?"=w202) -> ("error out"=w194:errorcluster)  [unwired: 9 in]
        n127 = call "Synchronize Module Events.vi"("error in"=w197, "Wait for Event Sync?"=w198) -> ("error out"=w195:errorcluster)  [unwired: 9 in]
        n128 = Merge Errors(w194, w195) -> (w193:errorcluster)
      }
      frame "Apps.Initialize4" {
        n129 = Unbundle By Name(w211) -> ("HW config.mux"=w210:string)
        n130 = Type Cast(type=refnum<visa-resource-name> refnum ("COMport name"), x=w210) -> (*(type *) &x=w208:refnum<visa-resource-name>)
        n131 = call "Start Module.vi"("error in (no error)"=w227, "COMport name"=w208) -> ("error out"=w224:errorcluster, "Wait for Event Sync?"=w223:bool, "MB 01 switches Module Broadcast Events"=w225:T11, "Module Was Already Running?"=w213:bool)  [unwired: 6 in]
        n132 = register-events(reference=w226, w225) -> (reference out=w219:refnum<event-registration>)  [unwired: 4 in, 1 out]
        n133 = local write "MB01 Module Running?"(w213) -> ()
        n134 = call "Synchronize Module Events.vi"("error in"=w224, "Wait for Event Sync?"=w223) -> ("error out"=w222:errorcluster)  [unwired: 9 in]
        n135 = call "Stop Module.vi"("error in"=w222, "Wait for Module to Stop? (F)"=TRUE) -> ("error out"=w220:errorcluster)  [unwired: 9 in]
        n136 = call "Start Module.vi"("error in (no error)"=w220, "COMport name"=w208) -> ("error out"=w216:errorcluster, "Wait for Event Sync?"=w215:bool, "MB 01 switches Module Broadcast Events"=w217:T11, "Module Was Already Running?"=w212:bool)  [unwired: 6 in]
        n137 = local write "MB01 Module Running?"(w212) -> ()
        n138 = register-events(reference=w219, w217) -> (reference out=w218:refnum<event-registration>)  [unwired: 4 in, 1 out]
        n139 = call "Synchronize Module Events.vi"("error in"=w216, "Wait for Event Sync?"=w215) -> ("error out"=w214:errorcluster)  [unwired: 9 in]
      }
      frame "Apps.Initialize Panel" {
        # "Initialize Panel - Initialize the appearance of the front panel here."
        n140 = disable-structure "Conditional Disable Structure" shown="Default" {
          disable-tunnel: ["development" w247 "Mac" "Linux"] -> w239
          frame condition #0 (active) {
          }
          frame condition #1 {
            n141 = Current VI's Path() -> (path=w248:path)
            n142 = while {
              border: w248 -> [_]
              tunnel: [w249] -> w247
              stop <- w253 continue-if-true
              # "this VI only \nworks in Windows"
              n143 = feedback #1() -> (w252:path)
              n144 = Strip Path(path=w252) -> (stripped path=w251:path)  [unwired: 1 out]
              n145 = feedback-in #1(w251) -> ()
              n146 = File/Directory Info(path=w251) -> (path out=w250:path, error out=w254:errorcluster)  [unwired: 1 in, 5 out]
              n147 = call <vilib>:"FileVersionInfo.vi"("error in (no error)"=w254, "Application Path in"=w250) -> ("error out"=w253:errorcluster, "File Version Info"=w249:string)  [unwired: 6 in, 2 out]
            }
          }
          frame condition #2 {
          }
          frame condition #3 {
          }
        }
        "version" <- w239
        n148 = control-ref of="Select CE14 eMIC module Module Instance"() -> (w233:refnum<vi>)
        n149 = Unbundle By Name(w243) -> ("Singleton Controls"=w242:refnum<vi>[])
        n150 = call "Update Select Module Ring.vi"("Select Module Ring Ref"=w233) -> ("Active Modules (Array)"=→"Active CE14 eMIC module Modules":string[], "New Module Ring Value"=w232:i32)  [unwired: 8 in, 1 out]
        n151 = property on="Property Node" class="Ring (strict)"(reference=w233, "Val(Sgnl)"=w232) -> ()  [unwired: 1 in, 2 out]
        n152 = for {
          tunnel: w242 -> [w258] mode=indexing
          n153 = property on="Property Node" class="Ctl"(reference=w258, "DisabledEnum"=T13."Disabled and Grayed Out" ("Disabled")) -> ()  [unwired: 1 in, 2 out]
        }
        n154 = local write "Switches Module Running?"(FALSE ("My Singleton Module Init?")) -> ()
        n155 = control-ref of="This VI"() -> (w235:refnum<vi>)
        n156 = call "Application Name--constant.vi"() -> ("Application Name"=w238:string)  [unwired: 11 in]
        n157 = property on="Property Node" class="VI"(reference=w235, "Front Panel.Title"=w238) -> (reference out=w237:refnum<vi>, error out=w245:errorcluster)  [unwired: 1 in]
        n158 = invoke class="VI" method="FP.Open"(reference=w237, error in=w245) -> ()  [unwired: 3 in, 5 out]
      }
      frame "Apps.UI Interlocks" {
        # "UI Interlocks - Disable the controls that would result in an error if the user selected them. In this case the Singleton Controls should be available only when the Singleton is running. The Cloneable Controls should be available if at least one clone instance is running."
        n159 = control-ref of="Select CE14 eMIC module Module Instance"() -> (w261:refnum<vi>)
        n160 = Unbundle By Name(w268) -> ("Singleton Controls"=w273:refnum<vi>[])
        n161 = Unbundle By Name(w268) -> ("Cloneable Controls"=w267:refnum<vi>[])
        n162 = call "Update Select Module Ring.vi"("Select Module Ring Ref"=w261) -> ("error out"=w259:errorcluster, "Active Modules (Array)"=w260:string[])  [unwired: 8 in, 1 out]
        n163 = local read "Switches Module Running?"() -> (w272:bool)
        n164 = Empty Array?(array=w260) -> (empty?=w277:bool)
        n165 = Not "Not Empty"(x=w277) -> (.not. x?=w266:bool)
        n166 = Select(t=T13."Enabled" ("Disabled"), s=w272, f=T13."Disabled and Grayed Out" ("Disabled")) -> (s? t:f=w274:T13)
        n167 = Select(t=T13."Enabled" ("Disabled"), s=w266, f=T13."Disabled and Grayed Out" ("Disabled")) -> (s? t:f=w271:T13)
        n168 = for {
          tunnel: w273 -> [w281] mode=indexing
          tunnel: w274 -> [w280]
          n169 = property on="Property Node" class="Ctl"(reference=w281, "DisabledEnum"=w280) -> ()  [unwired: 1 in, 2 out]
        }
        n170 = for {
          tunnel: w267 -> [w279] mode=indexing
          tunnel: w271 -> [w278]
          n171 = property on="Property Node" class="Ctl"(reference=w279, "DisabledEnum"=w278) -> ()  [unwired: 1 in, 2 out]
        }
      }
      frame "Apps.UI.Reinitiatize" {
        n172 = flat-sequence {
          tunnel: w285 -> [w289]
          tunnel: w282 -> [w296]
          tunnel: [w295] -> w283
          frame #0 {
            (unwired) u32 16711680  # NG
            (unwired) u32 6618880  # OK
            n173 = for {
              tunnel: w289 -> [w290] mode=indexing
              n174 = property class="ColBox"(reference=w290, "Value"=u32 10000536 ("DRV 1")) -> ()  [unwired: 1 in, 2 out]
            }
          }
          frame #1 {
            w294 = T8 {"Pass/Fail?"=FALSE, "AC Characteristic"={"Pass/Fail?"=FALSE, "Voltage"={"pass/fail?"=FALSE, "Measured Value"=0.0, "Upper Level"=0.0, "Lower Level"=0.0}, "Current"={"pass/fail?"=FALSE, "Measured Value"=0.0, "Upper Level"=0.0, "Lower Level"=0.0}, "Power factor"={"pass/fail?"=FALSE, "Measured Value"=0.0, "Upper Level"=0.0, "Lower Level"=0.0}, "Shorted Circuit"={"Pass/Fail?"=FALSE}}, "DC Characteristic"={"Pass/Fail?"=FALSE, "Voltage"={"pass/fail?"=FALSE, "Measured Value"=0.0, "Upper Level"=0.0, "Lower Level"=0.0}, "Current"={"pass/fail?"=FALSE, "Measured Value"=0.0, "Upper Level"=0.0, "Lower Level"=0.0}}}  # DUT cluster
            n175 = Initialize Array(w294, 60 ("dimension size")) -> (w292:T8[])
            n176 = Bundle By Name(cluster=w296, "DUT values"=w292) -> (w295:T7)
          }
        }
      }
      frame "Apps.Update Status" {
        # "Update Status - Display the latest status of the app in the Status indicator."
        n177 = Unbundle By Name(w302) -> ("Status"=→"Status":string)
      }
      frame "Apps.Wait for Event", Default {
        # "Wait for Event - Use an Event Structure to monitor the user interface for events that run different states of the state machine."
        n178 = event shown="[26] Timeout" {
          selector: w311 -> [w329 w352 w376 w391 _ _ _ _ _ _ _ _ _ _ _ _ _ _ _ _ _ _ _ _ _ _ _ _ _ _ _ _ _ _ _ _ _ _ _ _ _ _ _ _ _ _]
          dyn-events: [w328 w351 w360 w390 _ _ _ _ _ _ _ _ _ _ _ _ _ _ _ _ _ _ _ _ _ _ _ _ _ _ _ _ _ _ _ _ _ _ _ _ _ _ _ _ _ _] -> w310
          timeout: w304 -> [_ _ _ _ _ _ _ _ _ _ _ _ _ _ _ _ _ _ _ _ _ _ _ _ _ _ _ _ _ _ _ _ _ _ _ _ _ _ _ _ _ _ _ _ _ _]
          tunnel: [w323 w356 w357 w382 w399 w401 w415 w421 _ w427 w433 w441 w449 w455 _ _ _ w513 w521 _ _ _ w547 w553 w558 w562 w566 w571 w578 w583 w590 w596 w602 w614 w624 _ _ w642 _ _ _ _ w685 _ _ _] -> w312
          tunnel: [w326 w349 w359 w388 w395 w408 w413 w419 w424 w430 w436 w444 w452 w457 w469 w509 w512 w520 w528 w531 w537 w542 w549 w555 w560 w565 w569 w574 w580 w586 w592 w598 w604 w611 w621 w630 w637 w641 w645 w651 w662 w673 w678 w690 w696 w700] -> w308
          tunnel: w309 -> [w314 w342 w359 w378 w396 w407 w414 w420 w424 w430 w436 w444 w452 w457 w469 w509 w512 w518 w526 w532 w538 w543 w549 w555 w560 w565 w569 w574 w580 w586 w592 w598 w604 w611 w621 w630 w637 w641 w646 w652 w663 w674 w681 w691 w696 w700]
          tunnel: [App_States."Apps.Update Status" ("State") App_States."Apps.Update Status" ("State") App_States."Apps.Update Status" ("State") App_States."Apps.Update Status" ("State") App_States."Apps.Update Status" ("State") App_States."Apps.Update Status" ("State") App_States."Apps.Update Status" ("State") App_States."Apps.Update Status" ("State") App_States."Apps.Wait for Event" ("State") App_States."Apps.UI Interlocks" ("State") App_States."Apps.UI Interlocks" ("State") App_States."Apps.UI Interlocks" ("State") App_States."Apps.UI Interlocks" ("State") App_States."Apps.UI Interlocks" ("State") App_States."Apps.Wait for Event" ("State") App_States."Apps.Update Status" ("State") App_States."Apps.Wait for Event" ("State") App_States."Apps.Update Status" ("State") App_States."Apps.Update Status" ("State") App_States."Apps.Wait for Event" ("State") App_States."Apps.Wait for Event" ("State") App_States."Apps.Update Status" ("State") App_States."Apps.UI Interlocks" ("State") App_States."Apps.UI Interlocks" ("State") App_States."Apps.UI Interlocks" ("State") App_States."Apps.UI Interlocks" ("State") App_States."Apps.Wait for Event" ("State") App_States."Apps.UI Interlocks" ("State") App_States."Apps.UI Interlocks" ("State") App_States."Apps.UI Interlocks" ("State") App_States."Apps.UI Interlocks" ("State") App_States."Apps.UI Interlocks" ("State") App_States."Apps.UI Interlocks" ("State") App_States."Apps.UI Interlocks" ("State") App_States."Apps.UI Interlocks" ("State") App_States."Apps.UI Interlocks" ("State") App_States."Apps.UI Interlocks" ("State") App_States."Apps.UI Interlocks" ("State") App_States."Apps.Update Status" ("State") App_States."Apps.Update Status" ("State") App_States."Apps.Update Status" ("State") App_States."Apps.Update Status" ("State") App_States."Apps.UI Interlocks" ("State") App_States."Apps.UI Interlocks" ("State") App_States."Apps.Exit" ("State") App_States."Apps.Exit" ("State")] -> w307
          tunnel: w306 -> [_ _ _ _ _ _ _ _ _ w428 w434 w442 w450 _ _ _ _ _ _ _ _ _ w548 w554 w559 w563 w566 w572 w579 w584 w591 w597 w603 _ _ _ _ _ _ _ _ _ _ _ _ _]
          tunnel: w305 -> [_ _ _ _ _ _ _ _ _ _ _ _ _ _ _ _ _ _ _ _ _ _ _ _ _ _ _ _ _ _ _ _ _ _ _ _ _ _ _ _ _ _ _ _ _ _]
          tunnel: w304 -> [w324 w345 w370 w381 w393 w404 w410 w416 _ w429 w435 w443 w451 w458 w468 _ _ w515 w523 w529 w534 w539 w544 w550 w556 w561 w568 w570 w575 w581 w587 w593 w599 w609 w619 w626 w631 w638 w644 w649 w654 w665 w676 w686 w694 w698]
          tunnel: [w324 w345 w370 w381 w393 w404 w410 w416 "Time duration(ms)" w429 w435 w443 w451 w458 w468 -1 w511 w515 w523 w529 w534 w539 w544 w550 w556 w561 w568 w570 w575 w581 w587 w593 w599 w609 w619 w626 w631 w638 w644 w649 w654 w665 w676 w686 w694 w698] -> w303
          event "Start New Instance CE14 eMIC module Module": Value Change {
            n179 = event-data() -> ()  [unwired: 1 in, 1 out]
            n180 = Unbundle By Name(w314) -> ("HW config"=w313:T2)
            n181 = Unbundle By Name(w313) -> ("eMIC1"=w321:string, "eMIC2"=w320:string, "eMIC3"=w319:string, "eMIC4"=w318:string, "eMIC5"=w317:string, "eMIC6"=w316:string)
            n182 = Build Array(w321, w320, w319, w318, w317, w316) -> (w315:string[])
            n183 = for {
              N: 6 -> [_]
              tunnel: [w333] -> w323
              shift-right: [w339] -> w328
              shift-left: w329 -> [w340]
              tunnel: w315 -> [w331] mode=indexing
              n184 = Type Cast(type=refnum<visa-resource-name> refnum ("VISA resource name"), x=w331) -> (*(type *) &x=w330:refnum<visa-resource-name>)
              n185 = call "Start Module.vi"("VISA resource name"=w330) -> ("error out"=w337:errorcluster, "Wait for Event Sync?"=w335:bool, "CE14  Module Broadcast Events"=w336:T9, "Module ID"=w338:i32)  [unwired: 7 in]
              n186 = register-events(reference=w340, error in=w337, w336) -> (reference out=w339:refnum<event-registration>, error out=w334:errorcluster)  [unwired: 3 in]
              n187 = call "Synchronize Module Events.vi"("error in"=w334, "Wait for Event Sync?"=w335, "Module ID in"=w338) -> ("error out"=w333:errorcluster)  [unwired: 7 in, 1 out]
            }
            n188 = Bundle By Name(cluster=w314, "Status"="6 New instances of CE14 eMIC module Module started") -> (w326:T7)
          }
          event "Start Switches Module Module": Value Change {
            n189 = event-data() -> ()  [unwired: 1 in, 1 out]
            n190 = Unbundle By Name(w342) -> ("HW config.mux"=w341:string)
            n191 = Type Cast(type=refnum<visa-resource-name> refnum ("VISA resource name"), x=w341) -> (*(type *) &x=w343:refnum<visa-resource-name>)
            n192 = call "Start Module.vi"("VISA resource name"=w343) -> ("error out"=w355:errorcluster, "Wait for Event Sync?"=w353:bool, "Switches Module Broadcast Events"=w347:T10, "Module Was Already Running?"=w346:bool)  [unwired: 7 in]
            n193 = local write "Switches Module Running?"(w346) -> ()
            n194 = register-events(reference=w352, error in=w355, w347) -> (reference out=w351:refnum<event-registration>, error out=w354:errorcluster)  [unwired: 3 in]
            n195 = call "Synchronize Module Events.vi"("error in"=w354, "Wait for Event Sync?"=w353) -> ("error out"=w356:errorcluster)  [unwired: 9 in]
            n196 = Bundle By Name(cluster=w342, "Status"="New instance of Switches Module Module started") -> (w349:T7)
          }
          event "Start MB01 Module Module": Value Change {
            n197 = event-data() -> ()  [unwired: 1 in, 1 out]
            n198 = Unbundle By Name(w359) -> ("HW config.demux"=w358:string)
            n199 = Type Cast(type=refnum<visa-resource-name> refnum ("COMport name"), x=w358) -> (*(type *) &x=w361:refnum<visa-resource-name>)
            n200 = call "Start Module.vi"("COMport name"=w361) -> ("error out"=w373:errorcluster, "Wait for Event Sync?"=w372:bool, "MB 01 switches Module Broadcast Events"=w374:T11)  [unwired: 7 in, 1 out]
            n201 = register-events(reference=w376, error in=w373, w374) -> (reference out=w364:refnum<event-registration>, error out=w371:errorcluster)  [unwired: 3 in]
            n202 = call "Synchronize Module Events.vi"("error in"=w371, "Wait for Event Sync?"=w372) -> ("error out"=w369:errorcluster)  [unwired: 9 in]
            n203 = call "Stop Module.vi"("error in"=w369) -> ("error out"=w363:errorcluster)  [unwired: 10 in]
            n204 = call "Start Module.vi"("error in (no error)"=w363, "COMport name"=w361) -> ("error out"=w367:errorcluster, "Wait for Event Sync?"=w366:bool, "MB 01 switches Module Broadcast Events"=w368:T11)  [unwired: 6 in, 1 out]
            n205 = register-events(reference=w364, error in=w367, w368) -> (reference out=w360:refnum<event-registration>, error out=w365:errorcluster)  [unwired: 3 in]
            n206 = call "Synchronize Module Events.vi"("error in"=w365, "Wait for Event Sync?"=w366) -> ("error out"=w357:errorcluster)  [unwired: 9 in]
          }
          event "Start DMM Module Module": Value Change {
            n207 = event-data() -> ()  [unwired: 1 in, 1 out]
            n208 = Unbundle By Name(w378) -> ("HW config.DMM"=w377:string)
            n209 = Type Cast(type=refnum<visa-resource-name> refnum ("VISA resource name 2"), x=w377) -> (*(type *) &x=w379:refnum<visa-resource-name>)
            n210 = call "Start Module.vi"("VISA resource name 2"=w379) -> ("error out"=w383:errorcluster, "Wait for Event Sync?"=w385:bool, "DMM Module Broadcast Events"=w384:T12)  [unwired: 7 in, 1 out]
            n211 = register-events(reference=w391, error in=w383, w384) -> (reference out=w390:refnum<event-registration>, error out=w386:errorcluster)  [unwired: 3 in]
            n212 = call "Synchronize Module Events.vi"("error in"=w386, "Wait for Event Sync?"=w385) -> ("error out"=w382:errorcluster)  [unwired: 9 in]
            n213 = Bundle By Name(cluster=w378, "Status"="New instance of Switches Module Module started") -> (w388:T7)
          }
          event "Stop Switches Module Module": Value Change {
            n214 = event-data() -> ()  [unwired: 1 in, 1 out]
            n215 = call "Application Name--constant.vi"() -> ("Application Name"=w397:string)  [unwired: 11 in]
            n216 = call "Stop Module.vi"("Wait for Module to Stop? (F)"=TRUE, "Origin"=w397) -> ("error out"=w399:errorcluster)  [unwired: 9 in]
            n217 = Bundle By Name(cluster=w396, "Status"="Switches Module Module: Stopped" ("Message")) -> (w395:T7)
          }
          event "Stop CE14 eMIC module Module": Value Change {
            n218 = event-data() -> ()  [unwired: 1 in, 1 out]
            n219 = Unbundle By Name(w407) -> ("Module Ring Value"=w403:i32)
            n220 = Format Into String(format string="CE14 eMIC module Module instance %d: Stopped" ("Message"), w403) -> (resulting string=w405:string)  [unwired: 2 in, 1 out]
            n221 = call "Application Name--constant.vi"() -> ("Application Name"=w402:string)  [unwired: 11 in]
            n222 = call "Stop Module.vi"("Wait for Module to stop? (F)"=TRUE, "Origin"=w402, "Module ID"=w403) -> ("error out"=w401:errorcluster)  [unwired: 8 in]
            n223 = Bundle By Name(cluster=w407, "Status"=w405) -> (w408:T7)
          }
          event "Show Switches Module Module": Value Change {
            n224 = event-data() -> ()  [unwired: 1 in, 1 out]
            n225 = call "Show Panel.vi"() -> ("error out"=w415:errorcluster)  [unwired: 11 in]
            n226 = Bundle By Name(cluster=w414, "Status"="Showed Switches Module Module Panel" ("Message")) -> (w413:T7)
          }
          event "Hide Switches Module Module": Value Change {
            n227 = event-data() -> ()  [unwired: 1 in, 1 out]
            n228 = call "Hide Panel.vi"() -> ("error out"=w421:errorcluster)  [unwired: 11 in]
            n229 = Bundle By Name(cluster=w420, "Status"="Hid Switches Module Module Panel" ("Message")) -> (w419:T7)
          }
          event "Test": Value Change {
            n230 = event-data() -> ()  [unwired: 1 in, 1 out]
          }
          event "mux6-1(x1)": Value Change {
            n231 = event-data() -> ()  [unwired: 1 in, 1 out]
            n232 = call "inst.mux6_1(3wires).vi"("error in"=w428, "mux6_1(3wires)_encode"="mux6_1(3wires)_encode") -> ("error out"=w427:errorcluster)  [unwired: 9 in]
          }
          event "DMM input Selection": Value Change {
            n233 = event-data() -> ()  [unwired: 1 in, 1 out]
            n234 = call "DMM I 0.5_10.vi"("error in"=w434, "mux2-1(DMM I) encode"="mux2-1(DMM I) encode") -> ("error out"=w433:errorcluster)  [unwired: 9 in]
          }
          event "config DMM": Value Change {
            n235 = event-data() -> ()  [unwired: 1 in, 1 out]
            n236 = call "config channel.vi"("error in"=w442, "Detector Rate"="Detector Rate", "DCI range"="DCI range", "DCV range"="DCV range") -> ("error out"=w441:errorcluster)  [unwired: 7 in]
          }
          event "Read DCI, DCV  from DMM": Value Change {
            n237 = event-data() -> ()  [unwired: 1 in, 1 out]
            n238 = call "Read DCV_DCI.vi"("error in"=w450, "Sets to Display"="Sets to Display") -> ("error out"=w449:errorcluster, "DCI"=→"DCI":dbl, "DCV"=→"DCV":dbl)  [unwired: 6 in, 1 out]
          }
          event "Read ACI, ACV  from  eMIC(x6)": Value Change {
            n239 = event-data() -> ()  [unwired: 1 in, 1 out]
            n240 = call "FGV wait for 6 eMIC.vi"("Enum"=enum16{"Init", "count"}."Init") -> ()  [unwired: 10 in, 1 out]
            n241 = call "Read AC para.vi"("Module ID"=-1) -> ("error out"=w455:errorcluster)  [unwired: 10 in]
          }
          event User Event {
            w459 = T14 {"eMIC 1"={"ACV"=0.0, "ACI"=0.0, "pF"=0.0, "kW"=0.0}, "eMIC 2"={"ACV"=0.0, "ACI"=0.0, "pF"=0.0, "kW"=0.0}, "eMIC 3"={"ACV"=0.0, "ACI"=0.0, "pF"=0.0, "kW"=0.0}, "eMIC 4"={"ACV"=0.0, "ACI"=0.0, "pF"=0.0, "kW"=0.0}, "eMIC 5"={"ACV"=0.0, "ACI"=0.0, "pF"=0.0, "kW"=0.0}, "eMIC 6"={"ACV"=0.0, "ACI"=0.0, "pF"=0.0, "kW"=0.0}}  # eMICs cluster
            n242 = event-data() -> ("Module ID"=w463:i32, "eMIC response"=w462:T15[])  [unwired: 1 in]
            n243 = for {
              tunnel: w462 -> [w493] mode=indexing
              shift-right: [w489] -> w464
              shift-left: T1 {"ACV"=0.0, "ACI"=0.0, "pF"=0.0, "kW"=0.0} ("eMIC response") -> [w491]
              n244 = Unbundle By Name(w493) -> ("float"=w490:dbl, "Name"=w492:string)
              n245 = case shown="\"ACV\"" w492 {
                tunnel: w491 -> [w494 w497 w500 w503 w506]
                tunnel: w490 -> [_ w495 w498 w501 w505]
                tunnel: [w494 w496 w499 w502 w504] -> w489
                frame "False", Default {
                }
                frame "ACI" {
                  n246 = Bundle By Name(cluster=w497, "ACI"=w495) -> (w496:T1)
                }
                frame "kW" {
                  n247 = Bundle By Name(cluster=w500, "kW"=w498) -> (w499:T1)
                }
                frame "PF" {
                  n248 = Bundle By Name(cluster=w503, "pF"=w501) -> (w502:T1)
                }
                frame "ACV" {
                  n249 = Bundle By Name(cluster=w506, "ACV"=w505) -> (w504:T1)
                }
              }
            }
            "eMIC response" <- w464
            n250 = call "FGV wait for 6 eMIC.vi"("Enum"=enum16{"Init", "count"}."count") -> ()  [unwired: 10 in, 1 out]
            n251 = feedback #2(w459) -> (w460:T14)
            n252 = case shown="2" w463 {
              tunnel: w464 -> [_ w471 w474 w477 w480 w483 w486]
              tunnel: [w470 w472 w475 w478 w481 w484 w487] -> w461
              tunnel: w460 -> [w470 w473 w476 w479 w482 w485 w488]
              frame 0, Default {
              }
              frame 2 {
                n253 = Bundle By Name(cluster=w473, "eMIC 2"=w471) -> (w472:T14)
              }
              frame 3 {
                n254 = Bundle By Name(cluster=w476, "eMIC 3"=w474) -> (w475:T14)
              }
              frame 4 {
                n255 = Bundle By Name(cluster=w479, "eMIC 4"=w477) -> (w478:T14)
              }
              frame 5 {
                n256 = Bundle By Name(cluster=w482, "eMIC 5"=w480) -> (w481:T14)
              }
              frame 6 {
                n257 = Bundle By Name(cluster=w485, "eMIC 6"=w483) -> (w484:T14)
              }
              frame 1 {
                n258 = Bundle By Name(cluster=w488, "eMIC 1"=w486) -> (w487:T14)
              }
            }
            n259 = feedback-in #2(w461) -> ()
          }
          event "Pause": Value Change {
            n260 = event-data() -> ()  [unwired: 1 in, 1 out]
          }
          event "Again": Value Change {
            n261 = event-data() -> ()  [unwired: 1 in, 1 out]
            n262 = local read "Time duration(ms)"() -> (w511:i32)
          }
          event "Show CE14 eMIC module Module": Value Change {
            n263 = event-data() -> ()  [unwired: 1 in, 1 out]
            n264 = Unbundle By Name(w518) -> ("Module Ring Value"=w514:i32)
            n265 = Format Into String(format string="CE14 eMIC module Module instance %d: Panel Shown" ("Message"), w514) -> (resulting string=w516:string)  [unwired: 2 in, 1 out]
            n266 = call "Show Panel.vi"("Module ID"=w514) -> ("error out"=w513:errorcluster)  [unwired: 10 in]
            n267 = Bundle By Name(cluster=w518, "Status"=w516) -> (w520:T7)
          }
          event "Hide CE14 eMIC module Module": Value Change {
            n268 = event-data() -> ()  [unwired: 1 in, 1 out]
            n269 = Unbundle By Name(w526) -> ("Module Ring Value"=w522:i32)
            n270 = call "Hide Panel.vi"("Module ID"=w522) -> ("error out"=w521:errorcluster)  [unwired: 10 in]
            n271 = Format Into String(format string="CE14 eMIC module Module instance %d: Panel Hidden" ("Message"), w522) -> (resulting string=w524:string)  [unwired: 2 in, 1 out]
            n272 = Bundle By Name(cluster=w526, "Status"=w524) -> (w528:T7)
          }
          event "Select CE14 eMIC module Module Instance": Value Change {
            # "Store new selected Module ID value in shift register."
            n273 = event-data() -> ()  [unwired: 1 in, 1 out]
            n274 = Bundle By Name(cluster=w532, "Module Ring Value"="Select CE14 eMIC module Module Instance") -> (w531:T7)
          }
          event "Switches Module Module: Do Something": Value Change {
            # "Send \"Do Something\" request to Switches Module Module"
            n275 = event-data() -> ()  [unwired: 1 in, 1 out]
            n276 = Bundle By Name(cluster=w538, "Status"="\"Something\" button pressed in top-level application VI" ("\"Do Something Else\" button pressed")) -> (w537:T7)
          }
          event "Switches Module Module: Do Something Else": Value Change {
            # "Send \"Do Something Else\" request to Switches Module Module"
            n277 = event-data() -> ()  [unwired: 1 in, 1 out]
            n278 = Bundle By Name(cluster=w543, "Status"="\"Do Something Else\" numeric value changed in top-level application VI. New value: " ("\"Do Something Else\" button pressed")) -> (w542:T7)
          }
          event "DMM connect": Value Change {
            n279 = event-data() -> ()  [unwired: 1 in, 1 out]
            n280 = call "DMM init.vi"("error in"=w548, "VISA resource name"="DMM name") -> ("error out"=w547:errorcluster)  [unwired: 9 in]
          }
          event "Arduino connect": Value Change {
            n281 = event-data() -> ()  [unwired: 1 in, 1 out]
            n282 = call "MB01 Open.vi"("error in"=w554, "VISA resource name"="Arduino name") -> ("error out"=w553:errorcluster)  [unwired: 9 in]
          }
          event "M054 Close": Value Change {
            n283 = event-data() -> ()  [unwired: 1 in, 1 out]
            n284 = call "inst.Close.vi"("error in"=w559) -> ("error out"=w558:errorcluster)  [unwired: 10 in]
          }
          event "DMM Close": Value Change {
            n285 = event-data() -> ()  [unwired: 1 in, 1 out]
            n286 = call "DMM Close.vi"("error in"=w563) -> ("error out"=w562:errorcluster)  [unwired: 10 in]
          }
          event Timeout {
            n287 = event-data() -> ()  [unwired: 1 in, 1 out]
          }
          event "Arduino Close": Value Change {
            n288 = event-data() -> ()  [unwired: 1 in, 1 out]
            n289 = call "MB01 Close.vi"("error in"=w572) -> ("error out"=w571:errorcluster)  [unwired: 10 in]
          }
          event "M054 connect": Value Change {
            n290 = event-data() -> ()  [unwired: 1 in, 1 out]
            n291 = call "inst.Open.vi"("error in"=w579, "VISA resource name"="M054 name") -> ("error out"=w578:errorcluster)  [unwired: 9 in]
          }
          event "SC Enable": Value Change {
            n292 = event-data() -> ()  [unwired: 1 in, 1 out]
            n293 = call "SC enable.vi"("error in"=w584, "5V enable"="SC enable") -> ("error out"=w583:errorcluster)  [unwired: 9 in]
          }
          event "demux1-10(x6)": Value Change {
            n294 = event-data() -> ()  [unwired: 1 in, 1 out]
            n295 = call "demux1-10.vi"("error in"=w591, "demux1_10(x6)_encode"="demux1_10(x6)") -> ("error out"=w590:errorcluster)  [unwired: 9 in]
          }
          event "eMIC": Value Change {
            n296 = event-data() -> ()  [unwired: 1 in, 1 out]
            n297 = call "MB01_eMICs.vi"("error in"=w597, "Array"="eMIC (x6)") -> ("error out"=w596:errorcluster)  [unwired: 9 in]
          }
          event "mux10-1(x6)": Value Change {
            n298 = event-data() -> ()  [unwired: 1 in, 1 out]
            n299 = call "inst.mux10_1.vi"("error in"=w603, "mux10_1(x6)_encode"="mux10_1(x6)_encode") -> ("error out"=w602:errorcluster)  [unwired: 9 in]
          }
          event User Event {
            # "A new instance of CE14 eMIC module Module has broadcast that is has been initialized"
            n300 = event-data() -> ("Init?"=→"CE14 Module Running?":bool, "Info"=w613:string, "Module ID"=w610:i32)  [unwired: 1 in]
            n301 = control-ref of="Select CE14 eMIC module Module Instance"() -> (w608:refnum<vi>)
            n302 = local write "Status"(w613) -> ()
            n303 = call "Update Select Module Ring.vi"("Select Module Ring Ref"=w608) -> ("error out"=w606:errorcluster, "Active Modules (Array)"=w607:string[])  [unwired: 8 in, 1 out]
            n304 = local write "Active CE14 eMIC module Modules"(w607) -> ()
            n305 = disable-structure shown="Disabled" {
              disable-tunnel: [w617 w618] -> w614
              disable-tunnel: w606 -> [w616 w618]
              disable-tunnel: w610 -> [w615 _]
              frame Disabled {
                n306 = call "Show Panel.vi"("error in (no error)"=w616, "Module ID"=w615) -> ("error out"=w617:errorcluster)  [unwired: 9 in]
              }
              frame Enabled {
              }
            }
          }
          event User Event {
            # "Switches Module Module has broadcast that it has been initialized"
            n307 = event-data() -> ("Init?"=→"Switches Module Running?":bool, "Info"=w623:string)  [unwired: 1 in]
            n308 = local write "Status"(w623) -> ()
            n309 = disable-structure shown="Disabled" {
              disable-tunnel: [w625 _] -> w624
              frame Disabled {
                n310 = call "Show Panel.vi"() -> ("error out"=w625:errorcluster)  [unwired: 11 in]
              }
              frame Enabled {
              }
            }
          }
          event User Event {
            n311 = event-data() -> ("Init?"=→"DMM Module Running?":bool, "Info"=w628:string)  [unwired: 1 in]
            n312 = local write "Status"(w628) -> ()
          }
          event User Event {
            n313 = event-data() -> ("Init?"=→"MB01 Module Running?":bool, "Info"=w633:string)  [unwired: 1 in]
            n314 = Concatenate Strings(w633, "\r\n") -> (w632:string)
            n315 = local write "Status"(w632) -> ()
          }
          event User Event {
            # "Switches Module Module has broadcast its execution status"
            n316 = event-data() -> ("Running?"=w639:bool)  [unwired: 1 in]
            n317 = local write "Switches Module Running?"(w639) -> ()
            n318 = case shown="True" w639 {
              tunnel: [_ w643] -> w642
              frame False {
              }
              frame True {
                n319 = call "Show Panel.vi"() -> ("error out"=w643:errorcluster)  [unwired: 11 in]
              }
            }
          }
          event User Event {
            # "An instance of CE14 eMIC module Module has broadcast its status"
            n320 = event-data() -> ("Status"=w648:string)  [unwired: 1 in]
            n321 = Bundle By Name(cluster=w646, "Status"=w648) -> (w645:T7)
          }
          event User Event {
            # "Switches Module Module has broadcast its status"
            n322 = event-data() -> ("Status"=w653:string)  [unwired: 1 in]
            n323 = Bundle By Name(cluster=w652, "Status"=w653) -> (w651:T7)
          }
          event User Event {
            # "CE14 eMIC module Module had an error"
            n324 = event-data() -> ("Module Name"=w656:string, "Additional Information"=w659:string, "Error"=w664:errorcluster)  [unwired: 1 in]
            n325 = Unbundle By Name(w664) -> ("code"=w655:i32, "source"=w658:string)
            n326 = Format Into String(format string="Error code %d  Module: %s Additional Information: %s\nSource: %s", w655, w656, w659, w658) -> (resulting string=w657:string)  [unwired: 2 in, 1 out]
            n327 = Bundle By Name(cluster=w663, "Status"=w657) -> (w662:T7)
          }
          event User Event {
            # "Switches Module Module had an error"
            n328 = event-data() -> ("Module Name"=w667:string, "Additional Information"=w671:string, "Error"=w675:errorcluster)  [unwired: 1 in]
            n329 = Unbundle By Name(w675) -> ("code"=w666:i32, "source"=w670:string)
            n330 = Format Into String(format string="Error code %d Module: %s  Additional Information: %s\nSource: %s", w666, w667, w671, w670) -> (resulting string=w668:string)  [unwired: 2 in, 1 out]
            n331 = Bundle By Name(cluster=w674, "Status"=w668) -> (w673:T7)
          }
          event User Event {
            n332 = event-data() -> ("Origin"=w680:string)  [unwired: 1 in]
            n333 = Bundle By Name(cluster=w681, "Status"=w680) -> (w679:T7)
            n334 = control-ref of="Select CE14 eMIC module Module Instance"() -> (w684:refnum<vi>)
            n335 = call "Update Select Module Ring.vi"("Select Module Ring Ref"=w684) -> ("error out"=w685:errorcluster, "Active Modules (Array)"=w683:string[], "New Module Ring Value"=w677:i32)  [unwired: 8 in]
            n336 = Bundle By Name(cluster=w679, "Module Ring Value"=w677) -> (w678:T7)
            n337 = local write "Active CE14 eMIC module Modules"(w683) -> ()
          }
          event User Event {
            n338 = event-data() -> ("Origin"=w688:string)  [unwired: 1 in]
            n339 = local write "Switches Module Running?"(FALSE ("My Singleton Module Init?")) -> ()
            n340 = Concatenate Strings(w688, " Did Stop.") -> (w687:string)
            n341 = Bundle By Name(cluster=w691, "Status"=w687) -> (w690:T7)
          }
          event Panel Close? {
            # "Go to the 'Exit' state if the user tries to close the panel."
            n342 = event-data() -> ()  [unwired: 1 in, 1 out]
            n343 = event-data ("Event Filter Node")("Discard?"=TRUE) -> ()  [unwired: 1 in, 1 out]
          }
          event "Exit": Value Change {
            n344 = event-data() -> ()  [unwired: 1 in, 1 out]
          }
        }
      }
      frame "Apps.Exit" {
        w702 = TRUE  # Wait for Module to stop?
        w711 = TRUE  # Stop the VI
        # "Stop all modules launched"
        # "Exit - Exit the application."
        n345 = call "Application Name--constant.vi"() -> ("Application Name"=w703:string)  [unwired: 11 in]
        n346 = call "Stop Module.vi"("Wait for Module to Stop? (F)"=w702, "Origin"=w703) -> ("error out"=w713:errorcluster)  [unwired: 9 in]
        n347 = call "Stop Module.vi"("Wait for Module to Stop? (F)"=w702, "Origin"=w703) -> ("error out"=w708:errorcluster)  [unwired: 9 in]
        n348 = call "Stop Module.vi"("Wait for Module to Stop? (F)"=w702, "Origin"=w703) -> ("error out"=w707:errorcluster)  [unwired: 9 in]
        n349 = call "Stop Module.vi"("Wait for Module to stop? (F)"=w702, "Origin"=w703, "Module ID"=-1) -> ("error out"=w701:errorcluster)  [unwired: 8 in]
        n350 = Merge Errors(w701, w713, w708, w707) -> (w714:errorcluster)
      }
    }
    n351 = Or(x=w124, y=w120) -> (x .or. y?=w118:bool)
  }
  n352 = Unregister For Events(event registration refnum=w94) -> ()  [unwired: 1 in, 1 out]
  n353 = call <vilib>:"Simple Error Handler.vi"("error in (no error)"=w101) -> ("error out"=w100:errorcluster)  [unwired: 4 in, 4 out]
  n354 = disable-structure "Conditional Disable Structure" shown="Default" {
    disable-tunnel: w100 -> [_ _]
    frame condition #0 (active) {
    }
    frame condition #1 {
      # "Call Quit LabVIEW if running as a built application."
      n355 = Quit LabVIEW(quit? (T)=TRUE) -> ()
    }
  }
